vi "Lab2_1.vi"() -> ()   [LabVIEW 2021]
panel:
  in  "stop":bool
  in  "Keep Previous Location":bool
  out "2D Picture":picture
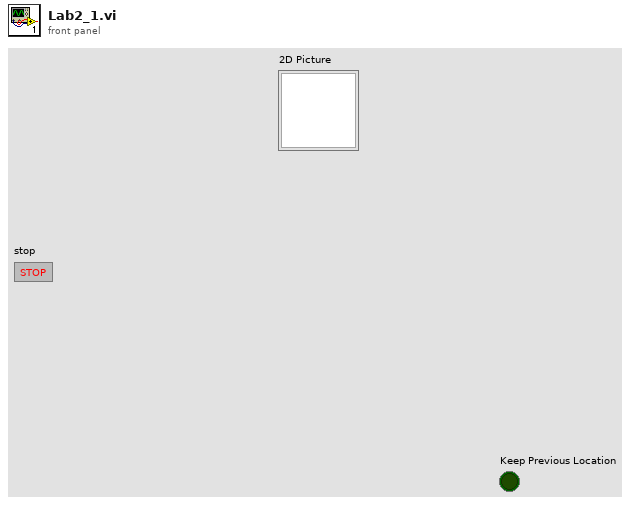
[diagram p1: front panel]
types:
  T1 = cluster{"Width":u16, "Style":enum32{"Solid", "Dash", "Dot", "DashDot", "DashDotDot"}}
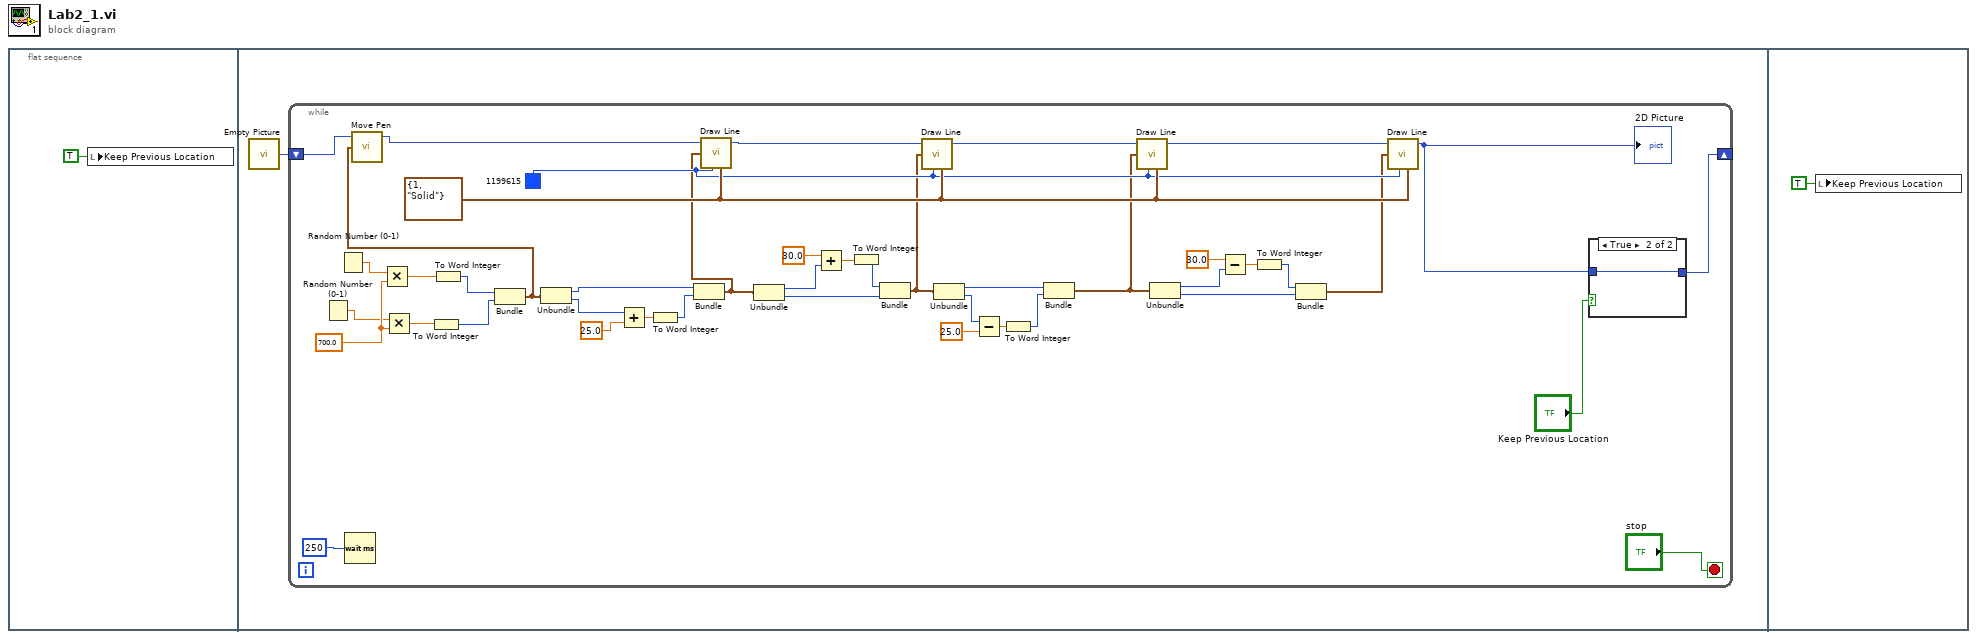
[diagram p0: block diagram]
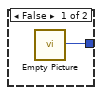
[diagram p2: hidden frame]
diagram:
  n1 = flat-sequence {
    frame #0 {
      n2 = local write "Keep Previous Location"(TRUE ("Keep Previous Location")) -> ()
    }
    frame #1 {
      n3 = call "Empty Picture"() -> ("empty picture"=w2:picture)
      n4 = while {
        shift-right: [w41] -> _
        shift-left: w2 -> [w46]
        stop <- "stop" stop-if-true
        w29 = u32 1199615 ("color(black)")
        w31 = T1 {"Width"=1, "Style"=enum."Solid"} ("pen")
        w39 = 700.0 ("y")
        n5 = Random Number (0-1)() -> (number: 0 to 1=w38:dbl)
        n6 = Random Number (0-1)() -> (number: 0 to 1=w37:dbl)
        n7 = Wait (ms)(milliseconds to wait=u32 250) -> ()  [unwired: 1 out]
        n8 = Multiply(x=w37, y=w39) -> (x*y=w36:dbl)
        n9 = Multiply(x=w38, y=w39) -> (x*y=w35:dbl)
        n10 = To Word Integer(number=w35) -> (16bit integer=w33:i16)
        n11 = To Word Integer(number=w36) -> (16bit integer=w34:i16)
        n12 = Bundle(w34, w33) -> (w32:cluster{i16, i16})  [unwired: 1 in]
        n13 = call <vilib>:"Move Pen.vi"("new position"=w32, "picture"=w46) -> ("new picture"=w45:picture)  [unwired: 3 in]
        n14 = Unbundle(w32) -> (w24:i16, w27:i16)
        n15 = Add(x=w27, y=25.0) -> (x+y=w26:dbl)
        n16 = To Word Integer(number=w26) -> (16bit integer=w25:i16)
        n17 = Bundle(w24, w25) -> (w23:cluster{i16, i16})  [unwired: 1 in]
        n18 = call <vilib>:"Draw Line.vi"("picture"=w45, "end point"=w23, "color(black)"=w29, "pen"=w31) -> ("new picture"=w44:picture)  [unwired: 5 in]
        n19 = Unbundle(w23) -> (w21:i16, w19:i16)
        n20 = Add(x=30.0, y=w21) -> (x+y=w20:dbl)
        n21 = To Word Integer(number=w20) -> (16bit integer=w18:i16)
        n22 = Bundle(w18, w19) -> (w17:cluster{i16, i16})  [unwired: 1 in]
        n23 = call <vilib>:"Draw Line.vi"("picture"=w44, "end point"=w17, "color(black)"=w29, "pen"=w31) -> ("new picture"=w43:picture)  [unwired: 5 in]
        n24 = Unbundle(w17) -> (w14:i16, w15:i16)
        n25 = Subtract(x=w15, y=25.0) -> (x-y=w4:dbl)
        n26 = To Word Integer(number=w4) -> (16bit integer=w13:i16)
        n27 = Bundle(w14, w13) -> (w12:cluster{i16, i16})  [unwired: 1 in]
        n28 = call <vilib>:"Draw Line.vi"("picture"=w43, "end point"=w12, "color(black)"=w29, "pen"=w31) -> ("new picture"=w42:picture)  [unwired: 5 in]
        n29 = Unbundle(w12) -> (w10:i16, w7:i16)
        n30 = Subtract(x=30.0, y=w10) -> (x-y=w9:dbl)
        n31 = To Word Integer(number=w9) -> (16bit integer=w8:i16)
        n32 = Bundle(w8, w7) -> (w6:cluster{i16, i16})  [unwired: 1 in]
        n33 = call <vilib>:"Draw Line.vi"("picture"=w42, "end point"=w6, "color(black)"=w29, "pen"=w31) -> ("new picture"=w40:picture)  [unwired: 5 in]
        "2D Picture" <- w40
        n34 = case shown="True" "Keep Previous Location" {
          tunnel: [w47 w48] -> w41
          tunnel: w40 -> [_ w48]
          frame False {
            n35 = call "Empty Picture"() -> ("empty picture"=w47:picture)
          }
          frame True {
          }
        }
      }
    }
    frame #2 {
      n36 = local write "Keep Previous Location"(TRUE ("Keep Previous Location")) -> ()
    }
  }
